vi "gpib.vi"() -> ()   [LabVIEW 2015]
doc: "This sub-VI reads and interprets a wave from the LeCroy oscilloscope. version a.0\n SubVI: \"LC 9400 Read\" reads and interprets a wave from the oscilloscope. First this subVI reads and parses the wave descriptor. Then it uses this information to read the wave from the scope, and finally, it converts the binary wave data into an amplitude (voltage) array, t-offset, and t-increment.\n The t-offset is the time between the first value of the array and the trigger point. It can be used to plot the wave relative to the trigger point (The trigger point is at time=0 seconds.).\n This subVI allows the user to pick both the part of the wave to read, and the number of points to read. The wave can be read either from the beginning to the end (whole wave), the trigger position to the end (trig-> end), or the beginning of the screen to the end (displayed - this is the part of the wave that is shown on the scope's screen). Also, the number of points that can be read ranges from 0 to 32000. Points will be skipped in order to come out with an array of the desired length. Example: If 1000 points of the whole wave (32000 points) are to be read then only every 32nd point (the other 31 are skipped) is read from the scope.\n Note1: When reading from the trigger to the end, or just the\n displayed wave, 32000 points can't always be read. \n Note2: The wave cannot be read in interleaved sampling or in sequence\n trigger mode. Doing a read in one of these modes will result in\n an incorrect data array.\n\nDefaults, Ranges, and Numeric codes for controls.\n\n\n SubVI: \"LC 9400 Read\"\n *Number of points to read: Numeric Default: 1000 pts\n Range: 0 to 32000 pts\n *Wave to read: Default: channel 1\n 0=ch1, 1=ch2, 2=memory C, 3=memory D\n *Part of wave to read: Default: Whole\n 0=whole, 1= trigger to end, 2= displayed\n\n * Indicates controls that are connected to the connector pane."
panel:
  out "data":string
  in  "GPIB Address":string="4"
  in  "Samples Taken (full displays)":i32=100 caption="Numeric"
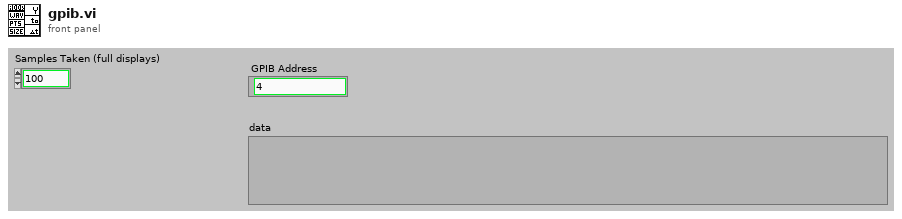
[diagram p1: front panel]
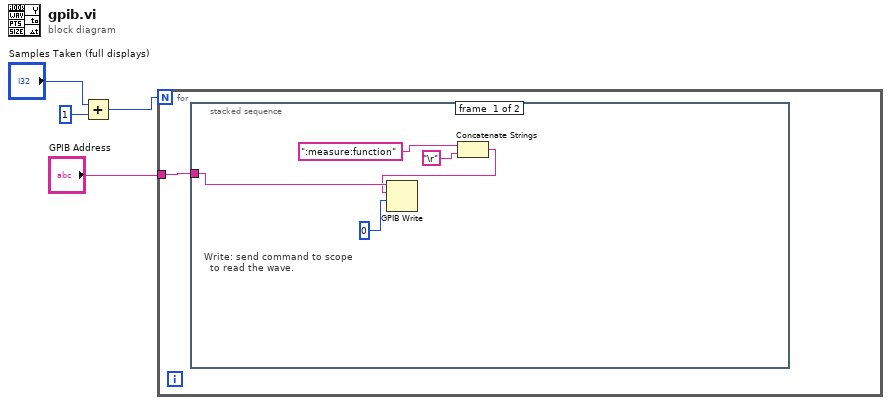
[diagram p0: block diagram]
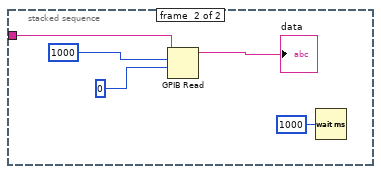
[diagram p2: hidden frame]
diagram:
  n1 = Add(x="Samples Taken (full displays)", y=1) -> (x+y=w2:i32)
  n2 = for {
    N: w2 -> [_]
    tunnel: "GPIB Address" -> [w5]
    n3 = stacked-sequence {
      tunnel: w5 -> [w9 w14]
      frame #0 {
        # "Write: send command to scope\n  to read the wave."
        n4 = Concatenate Strings(":measure:function" ("data"), "\r") -> (w8:string)
        n5 = GPIB Write(0:w9, 1:w8, 2:0) -> ()  [unwired: 2 in, 2 out]
      }
      frame #1 {
        n6 = GPIB Read(0:w14, 1:1000 ("byte count"), 2:0) -> (5:→"data":string)  [unwired: 2 in, 2 out]
        n7 = Wait (ms)(milliseconds to wait=u32 1000) -> ()  [unwired: 1 out]
      }
    }
  }
